vi "Nodes to UIDs.vi"(10 "cluster":T1, 11 "All Objects[]":refnum<vi>[](array[refnum])) -> (2 "Nodes":T1={"Depth"=0, "Top"=0, "Left"=0, "Frame index"=0, "Struct"=-1, "Object Class Name"="", "Object UID"=-1, "Label Visible"=FALSE, "Object Label"="", "SD Label Visible"=FALSE, "Object SD Label"="", "Frame Name"="", "Diag UID"=-1, "Owner Class Name"="", "Owner UID"=-1, "Diag Struct"=[], "Parent Struct"=0, "Diag UIDs"=[], "Tree Name"="", "Diag Ref"=refnum, "Owner Classes"=[], "Owner"=refnum, "Owner UIDs"=[], "Tag Indent"=0, "Tag Value"=0, "Child Tag"=""})   [LabVIEW 2023, in "VIDoc Parsing.lvlib" / "Structure Reporter.lvlib"]
uses:
  Structure Reporter.lvlib
  Structure Result 2.ctl
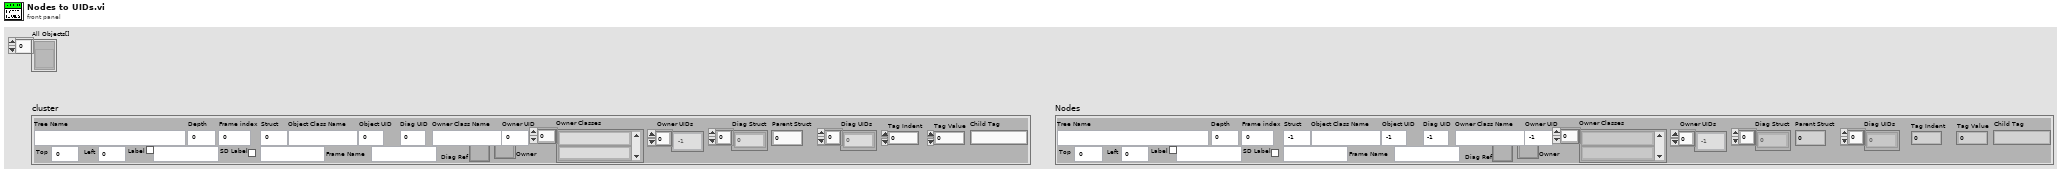
[diagram p1: front panel]
types:
  T1 = typedef "VIDoc Parsing.lvlib/Structure Reporter.lvlib/Structure Result 2.ctl" = cluster{"Depth":i32, "Top":i32, "Left":i32, "Frame index":i32, "Struct":i32, "Object Class Name":string, "Object UID":i32, "Label Visible":bool, "Object Label":string, "SD Label Visible":bool, "Object SD Label":string, "Frame Name":string, "Diag UID":i32, "Owner Class Name":string, "Owner UID":i32, "Diag Struct":i32[], "Parent Struct":i32, "Diag UIDs":i32[], "Tree Name":string, "Diag Ref":refnum<vi>, "Owner Classes":string[], "Owner":refnum<vi>, "Owner UIDs":i32[], "Tag Indent":i32, "Tag Value":i32, "Child Tag":string}
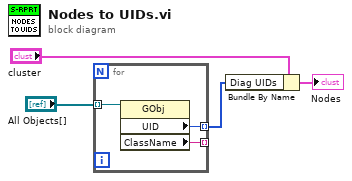
[diagram p0: block diagram]
diagram:
  n1 = for {
    tunnel: "All Objects[]" -> [w7] mode=indexing
    tunnel: [w6] -> w1 mode=indexing
    tunnel: [w5] -> _ mode=indexing
    n2 = property class="GObj"(reference=w7) -> ("UID"=w6:i32, "ClassName"=w5:string)  [unwired: 1 in, 2 out]
  }
  n3 = Bundle By Name(cluster="cluster", "Diag UIDs"=w1) -> (→"Nodes":T1)
